vi "Init.vi"(8 "error in (no error)":errorcluster, 10 "Size":i32, 11 "Prime_Sieve in":refnum<class "Prime_Sieve.lvclass">) -> (0 "error out":errorcluster, 3 "Prime_Sieve out":refnum<class "Prime_Sieve.lvclass">)   [LabVIEW 2025, in "Prime_Sieve.lvclass"]
uses:
  Prime_Sieve.lvclass
  Prime_Sieve.lvclass/Prime_Sieve.ctl
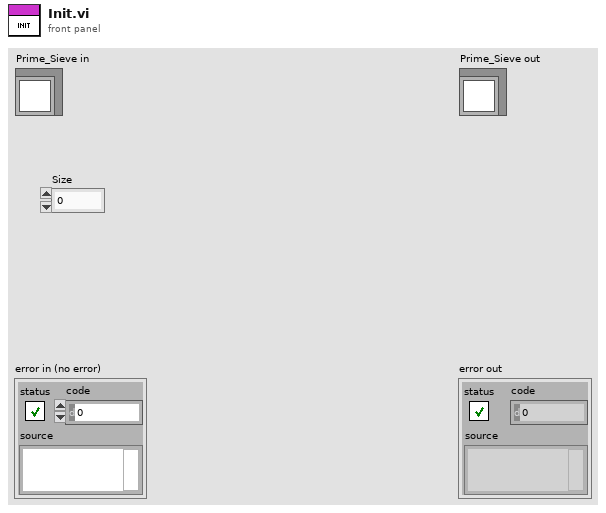
[diagram p1: front panel]
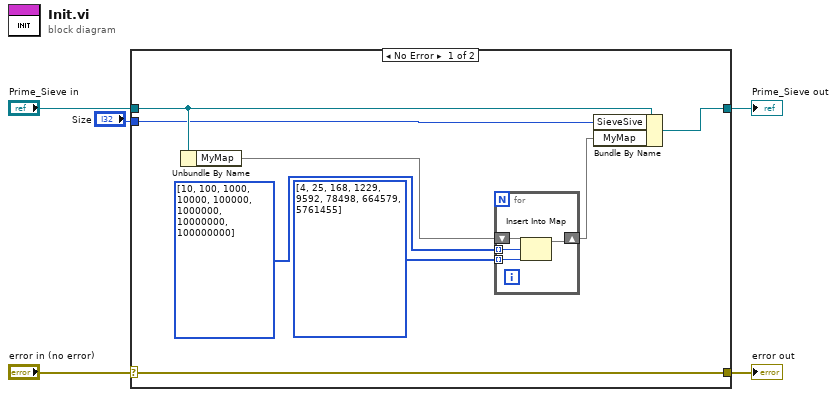
[diagram p0: block diagram]
diagram:
  n1 = case shown="No Error" "error in (no error)" {
    selector: "error in (no error)" -> [w13 w19]
    tunnel: [w13 w19] -> w4
    tunnel: [w12 w18] -> w2
    tunnel: "Prime_Sieve in" -> [w11 w18]
    tunnel: "Size" -> [w6 _]
    frame No Error {
      n2 = Unbundle By Name(w11) -> ("MyMap"=w10:map{i64, i32})
      n3 = for {
        shift-right: [w16] -> w7
        shift-left: w10 -> [w17]
        tunnel: i64[] [10, 100, 1000, 10000, 100000, 1000000, 10000000, 100000000] -> [w15] mode=indexing
        tunnel: i32[] [4, 25, 168, 1229, 9592, 78498, 664579, 5761455] -> [w14] mode=indexing
        n4 = Insert Into Map(map in=w17, key=w15, value=w14) -> (map out=w16:map{i64, i32})  [unwired: 2 out]
      }
      n5 = Bundle By Name(cluster=w11, "SieveSive"=w6, "MyMap"=w7) -> (w12:refnum<class "Prime_Sieve.lvclass">)
    }
    frame Error {
    }
  }
  "error out" <- w4
  "Prime_Sieve out" <- w2
